vi "2014 Target Detection.vi"() -> ()   [LabVIEW 2013]
uses:
  <vilib>/Rock Robotics/WPI/Camera/WPI_CameraSettings Read MJPG.ctl
  <vilib>/Rock Robotics/WPI/Camera/WPI_CameraImageSize.ctl
  TargetType.ctl
panel:
  in  "Instructions:":string="Images:\nUse the tab immediately below to choose the image source. Update the camera settings or the image directory so that you have images or video to test with.\n\nCalibration:\nYou can update Color Component ranges directly, or by clicking and drawing a line on the colored strip in the Image control. The Std Dev multipliers and where the strip is drawn determine the calibration values.\n\nUse Debugging tab to view the result of the color range threshold .\n\nArea Size LImit is used to ignore objects too small or far away to care about.\n\nThe Details tab contains score details for each target and subObject.\n\nCamera Type is used to select lens angles for distance calculation.\n\nVertical strips with no adjacent horizontal strip are identified as \"not hot\" and marked in blue.\nThe numeric scores indicate represent aspect ratio and rectangularity.\n\nWhen both strips are near enough, the pair is identified as \"hot\" and marked in green. Scores\nindicate the left, right, ratio of widths, and vertical positioning.\n\nAny score that falls below cutoff is drawn in red and bounding box is drawn in red."
  in  "Std Devs":cluster{"Hue":dbl, "Sat":dbl, "Val":dbl}={"Hue"=4.0, "Sat"=6.0, "Val"=4.0}
  in  "Area Size Limit %":dbl=0.06 format="%#_13g"
  in  "Camera Type":enum16{"206", "1011", "1013"}(ring)=enum."1013"
  out "loop time ms":u32=29
  in  "Score Cutoff":dbl(slide)=50.467289719626166 scale=0.0..100.0
  in  "Color Components":T1={"Hue"={110.68181610107422, 142.68181610107422}, "Sat"={230.14772033691406, 255.0}, "Val"={238.89772033691406, 255.0}} {"Val" scale=0.0..255.0; "Sat" scale=0.0..255.0; "Hue" scale=0.0..255.0 scale format="%#_3g"}
  out "Error":bool
  in  "Image Source":enum32{"Files", "Camera"}(tab)
  in  "List of image files":i32(listbox)=18
  in  "Image Directory":path=path "C:/Users/Bowers/Desktop"
  in  "Camera Settings":T2={"fps"=15, "compression"=5, "Image Size"=enum."320x240"}
  in  "Camera IP":string="10.00.00.11"
  in  "Tabbed Info":enum32{"Debugging", "Details"}(tab)
  out "Mask":T4(plugin-control)
  out "Target Info":T6(array[cluster])
  out "Image":T4(plugin-control)
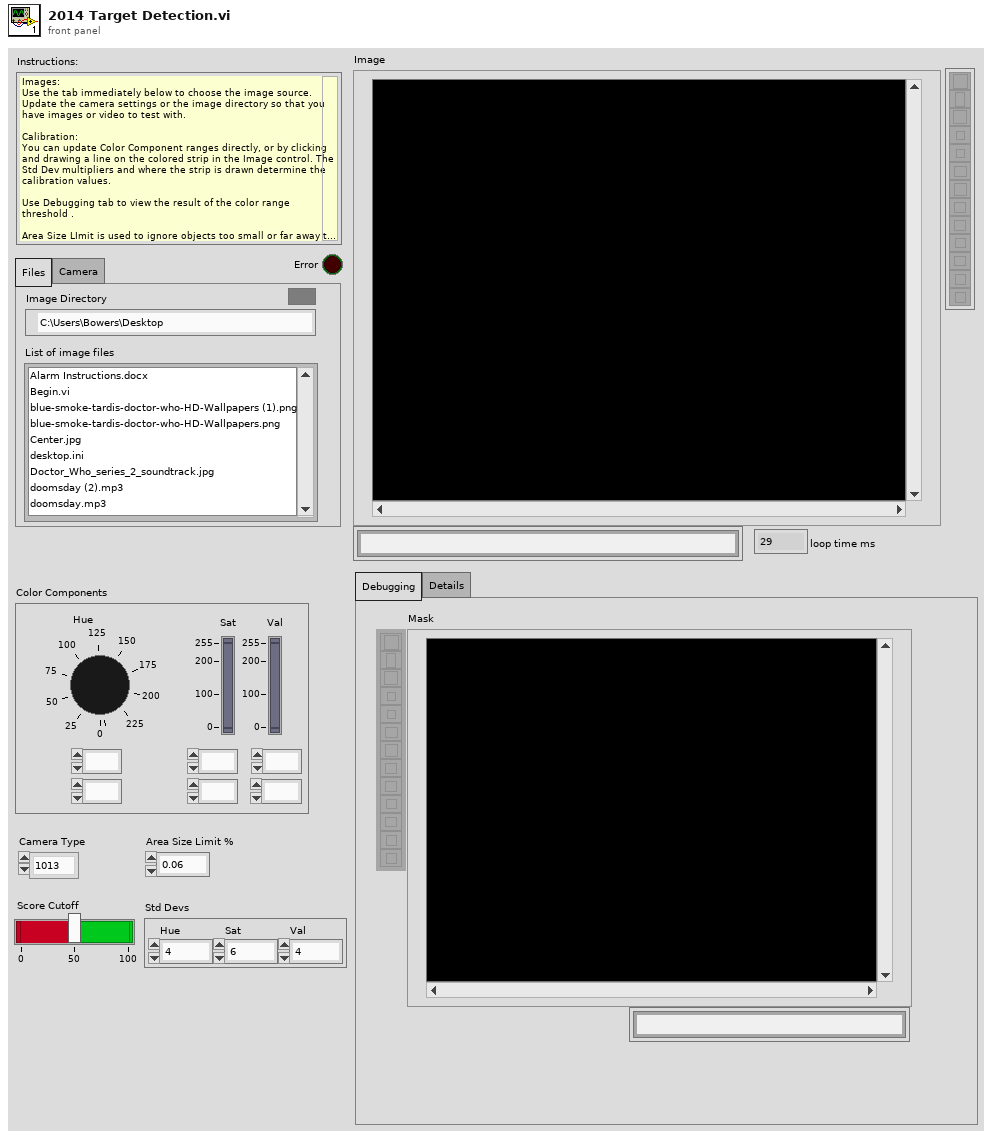
[diagram p1: front panel]
types:
  T1 = cluster{"Hue":cluster{dbl, dbl}, "Sat":cluster{dbl, dbl}, "Val":cluster{dbl, dbl}}
  T2 = typedef "WPI_CameraSettings Read MJPG.ctl" = cluster{"fps":i32, "compression":i32, "Image Size":T3}
  T3 = typedef "WPI_CameraImageSize.ctl" = enum16{"640x480", "320x240", "160x120"}
  T4 = typedef "IMAQ Image.ctl" = refnum<image>
  T5 = typedef "TargetType.ctl" = enum16{"Not Hot", "Hot"}
  T6 = cluster{"Scores":cluster{"Total":dbl, "Left":dbl, "Right":dbl, "Ratio":dbl, "Vertical":dbl, "index":i32, "State":T5}, "Verticals":cluster{"Horizontal?":bool, "Aspect Score":dbl, "Rect Score":dbl, cluster{"Left":dbl, "Top":dbl, "Right":dbl, "Bottom":dbl}, "Equiv H":dbl, "Equiv V":dbl}, "Horizontals":cluster{"Horizontal?":bool, "Aspect Score":dbl, "Rect Score":dbl, cluster{"Left":dbl, "Top":dbl, "Right":dbl, "Bottom":dbl}, "Equiv H":dbl, "Equiv V":dbl}, "Distance ft":dbl, "Center":cluster{"X":dbl, "Y":dbl}}[]
  T7 = typedef "Image Type" = u32
  T8 = cluster{"Horizontal":bool, "Aspect Score":dbl, "Rect Score":dbl, cluster{"Left":dbl, "Top":dbl, "Right":dbl, "Bottom":dbl}, "Equiv H":dbl, "Equiv V":dbl}[]
  T9 = cluster{cluster{dbl, dbl}, cluster{dbl, dbl}, cluster{dbl, dbl}}
  T10 = cluster{"Scores":cluster{"Total":dbl, "Left":dbl, "Right":dbl, "Ratio":dbl, "Vertical":dbl, "index":i32, "State":T5}, "Verticals":cluster{"Horizontal?":bool, "Aspect Score":dbl, "Rect Score":dbl, cluster{"Left":dbl, "Top":dbl, "Right":dbl, "Bottom":dbl}, "Equiv H":dbl, "Equiv V":dbl}, "Horizontals":cluster{"Horizontal?":bool, "Aspect Score":dbl, "Rect Score":dbl, cluster{"Left":dbl, "Top":dbl, "Right":dbl, "Bottom":dbl}, "Equiv H":dbl, "Equiv V":dbl}, "Validated":bool}[]
  T11 = cluster{"Scores":cluster{"Total":dbl, "Left":dbl, "Right":dbl, "Ratio":dbl, "Vertical":dbl, "index":i32, "State":T5}, "Verticals":cluster{"Horizontal?":bool, "Aspect Score":dbl, "Rect Score":dbl, cluster{"Left":dbl, "Top":dbl, "Right":dbl, "Bottom":dbl}, "Equiv H":dbl, "Equiv V":dbl}, "Horizontals":cluster{"Horizontal?":bool, "Aspect Score":dbl, "Rect Score":dbl, cluster{"Left":dbl, "Top":dbl, "Right":dbl, "Bottom":dbl}, "Equiv H":dbl, "Equiv V":dbl}, "Distance (ft)":dbl, "Target Center (-1 to 1)":cluster{"X":dbl, "Y":dbl}}[]
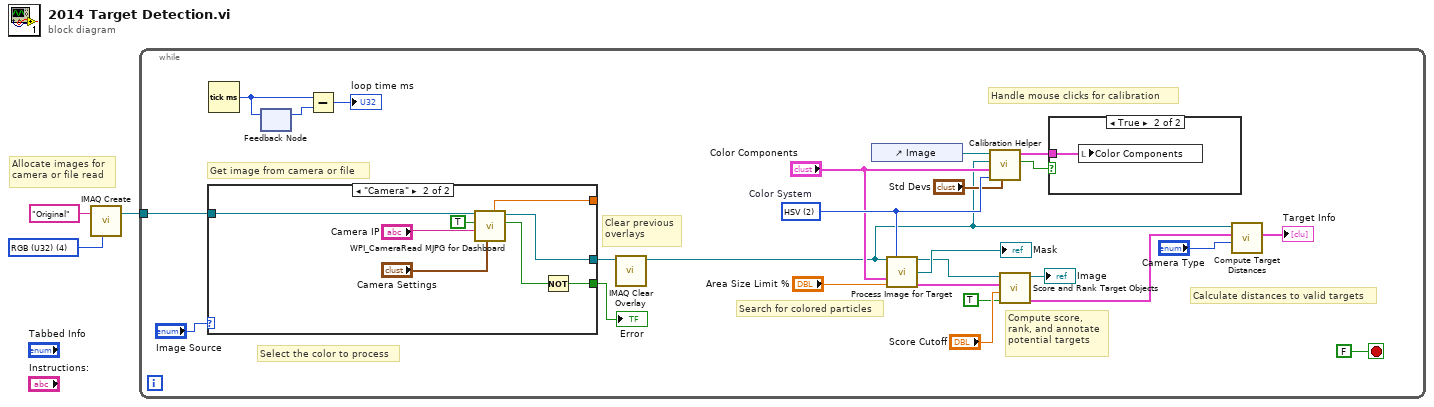
[diagram p0: block diagram]
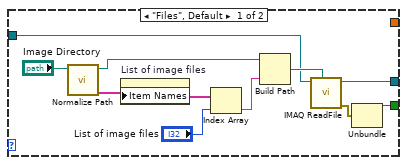
[diagram p3: hidden frame]
diagram:
  w3 = T7 4 items=["Grayscale (U8)", "Grayscale (I16)", "Grayscale (SGL)", "Complex (CSG)", "RGB (U32)", "HSL (U32)", "RGB (U64)", "Grayscale (U16)"] ("Image Type")
  # "Allocate images for\ncamera or file read"
  n1 = call "IMAQ Create"("Image Name"="Original", "Image Type"=w3) -> ("New Image"=w1:T4)  [unwired: 3 in, 1 out]
  n2 = while {
    tunnel: w1 -> [w25]
    stop <- FALSE stop-if-true
    w10 = u16 2 items=["RGB", "HSL", "HSV", "HSI"]  # Color System
    # "Clear previous\noverlays"
    # "Calculate distances to valid targets"
    # "Search for colored particles"
    # "Handle mouse clicks for calibration"
    # "Compute score,\nrank, and annotate\npotential targets"
    # "Select the color to process"
    # "Get image from camera or file"
    n3 = case shown="\"Camera\"" "Image Source" {
      tunnel: [w36 w46] -> w28
      tunnel: w25 -> [w35 w47]
      tunnel: [w33 w41] -> w24
      tunnel: [_ w40] -> _
      frame "Files", Default {
        n4 = call "Normalize Path.vi"("Image Directory"="Image Directory") -> ("Filenames"=w31:string[], "Path"=w30:path)  [unwired: 9 in]
        n5 = property on="List of image files" class="LstBox (strict)"("Item Names"=w31) -> ()  [unwired: 2 in, 2 out]
        n6 = Index Array(array=w31, index="List of image files") -> (element=w38:string)
        n7 = Build Path(base path=w30, name or relative path=w38) -> (appended path=w37:path)
        n8 = call "IMAQ ReadFile"("File Path"=w37, "Image"=w35) -> ("error out"=w34:errorcluster, "Image Out"=w36:T4)  [unwired: 5 in, 3 out]
        n9 = Unbundle(w34) -> ("status"=w33:bool)  [unwired: 2 out]
      }
      frame "Camera" {
        n10 = call <vilib>:"WPI_CameraRead MJPG for Dashboard.vi"("Camera Settings"="Camera Settings", "Camera IP"="Camera IP", "Enable"=TRUE, "Refnum in"=w47) -> ("Active"=w43:bool, "Refnum out"=w46:T4, "Bandwidth (Mbps)"=w40:dbl)  [unwired: 4 in, 1 out]
        n11 = Not(x=w43) -> (.not. x?=w41:bool)
      }
    }
    "Error" <- w24
    n12 = Tick Count (ms)() -> (millisecond timer value=w23:u32)
    n13 = feedback #1() -> (w22:u32)  [unwired: 1 in]
    n14 = feedback-in #1(w23) -> ()
    n15 = Subtract(x=w23, y=w22) -> (x-y=→"loop time ms":u32)
    n16 = call "IMAQ Clear Overlay"("Image"=w28) -> ("Image Out"=w5:T4)  [unwired: 9 in, 1 out]
    n17 = control-ref of="Image"() -> (w11:refnum<vi>)
    n18 = call "Process Image for Target.vi"("Src Image"=w5, "Color Mode"=w10, "Color Components"="Color Components", "Area Cutoff %"="Area Size Limit %") -> ("Src Image Out"=w18:T4, "Threshold"=→"Mask":T4, "Particles"=w15:T8)  [unwired: 9 in]
    n19 = call "Calibration Helper.vi"("Std Devs"="Std Devs", "Color Mode"=w10, "Color Components"="Color Components", "Image"=w5, "Image Ctl Refnum"=w11) -> ("Changed"=w6:bool, "output color"=w8:T9)  [unwired: 5 in]
    n20 = call "Score and Rank Target Objects.vi"("Annotate"=TRUE, "Score Limit"="Score Cutoff", "Particles"=w15, "Image in"=w18) -> ("Target Info"=w14:T10, "Annotated Image"=→"Image":T4)  [unwired: 6 in]
    n21 = case shown="True" w6 {
      tunnel: w8 -> [_ w29]
      frame False {
      }
      frame True {
        n22 = local write "Color Components"(w29) -> ()
      }
    }
    n23 = call "Compute Target Distances.vi"("Camera Type"="Camera Type", "Target Info"=w14, "Image in"=w5) -> ("Target Info"=→"Target Info":T11)  [unwired: 6 in, 2 out]
  }
